vi "1byte.vi"() -> ()   [LabVIEW 2020]
panel:
  out "Actual Bitrate kHz":i32=1000
  out "error out":errorcluster
  in  "SCLK (kHz)":i32=2000 min=0
  out "Cheetah Handle":i32
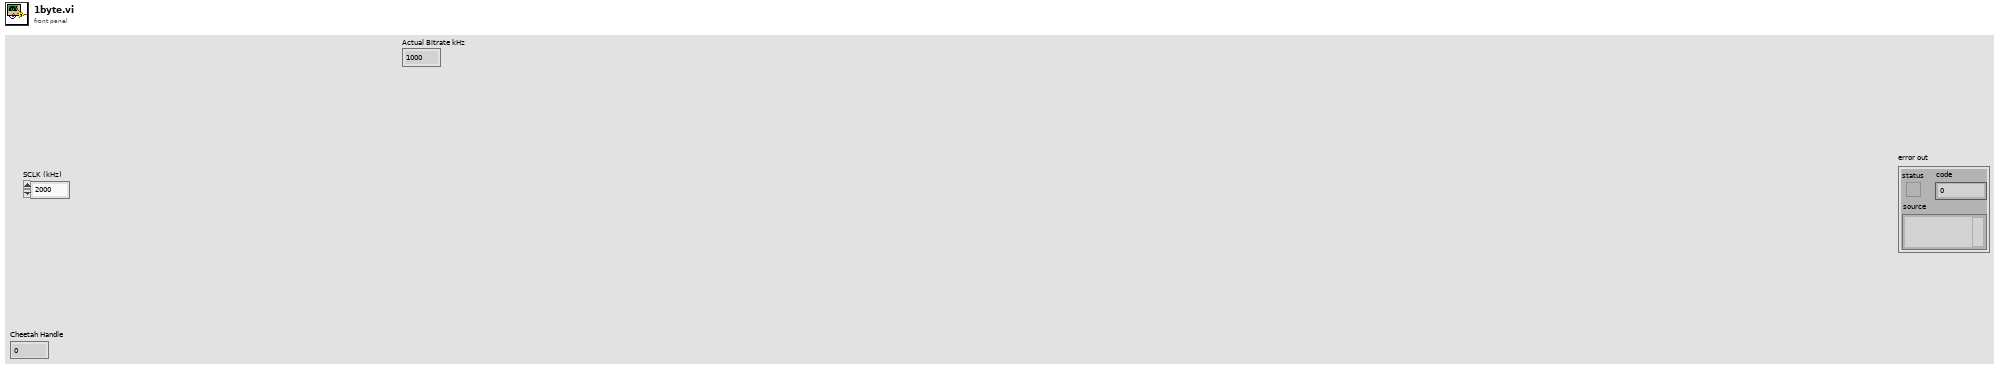
[diagram p1: front panel]
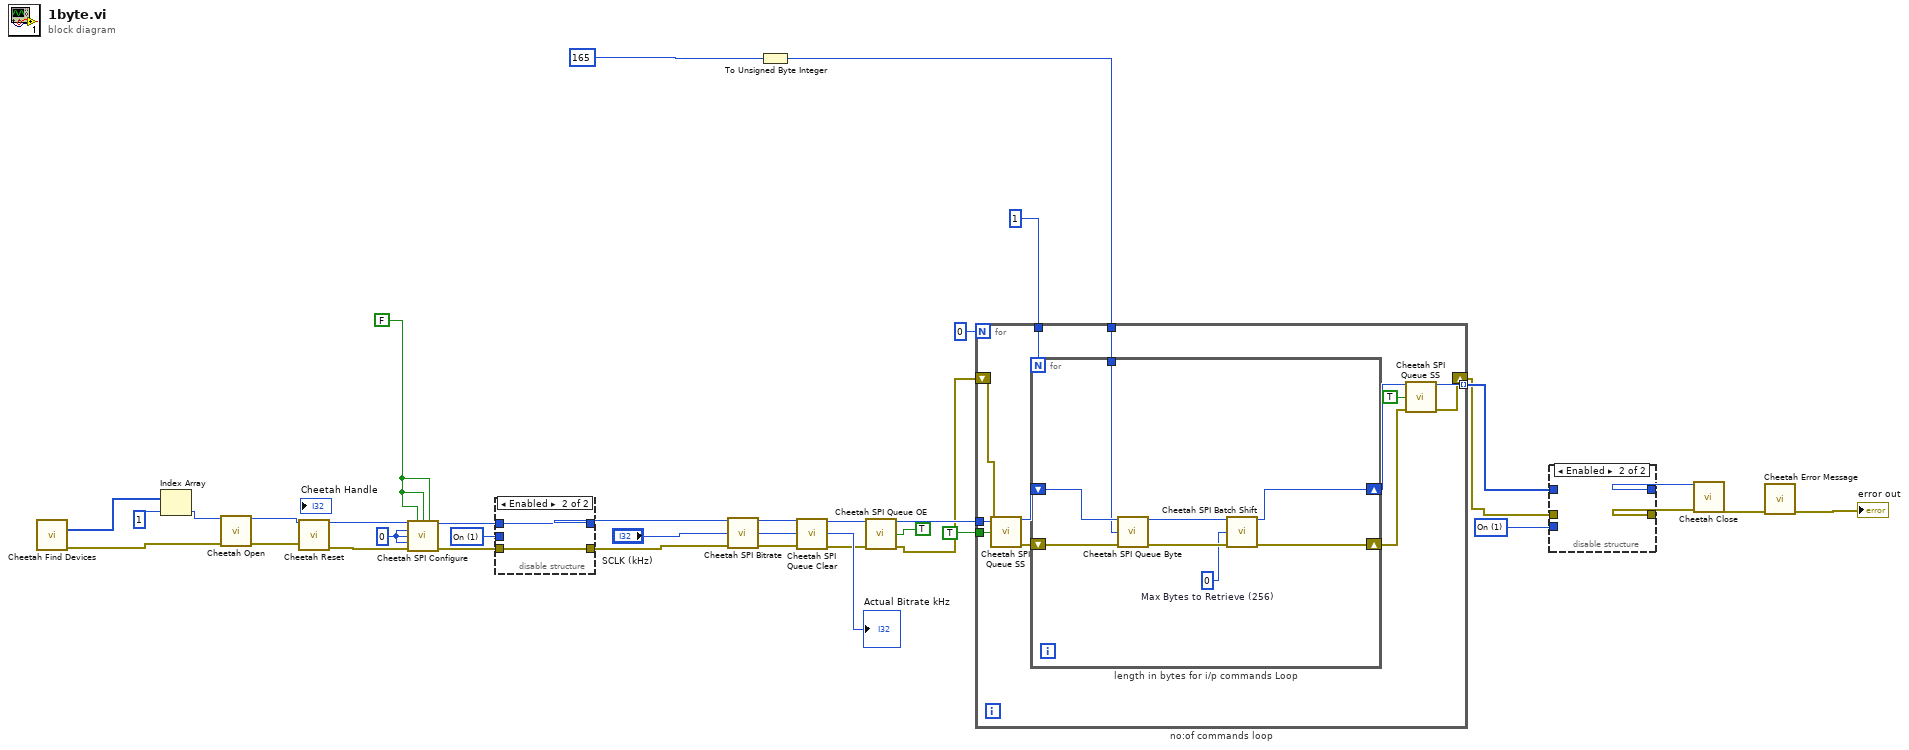
[diagram p0: block diagram]
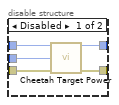
[diagram p2: hidden frame]
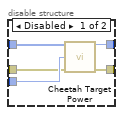
[diagram p3: hidden frame]
diagram:
  w1 = u16 1 items=["Off", "On", "Query"] ("Requested Configuration (2: Query)")
  w22 = u16 1 items=["Off", "On", "Query"] ("Requested Configuration (2: Query)")
  w33 = FALSE
  w34 = 0
  n1 = call <instrlib>:"Cheetah Find Devices.vi"() -> ("Ports"=w35:u16[], "error out"=w10:errorcluster)  [unwired: 13 in, 1 out]
  n2 = Index Array(array=w35, index=1) -> (element=w9:u16)
  n3 = call <instrlib>:"Cheetah Open.vi"("Port Number (0)"=w9, "error in (no error)"=w10) -> ("Cheetah Handle"=w6:i32, "error out"=w7:errorcluster)  [unwired: 12 in]
  n4 = call <instrlib>:"Cheetah Reset.vi"("Cheetah Handle (0)"=w6, "error in (no error)"=w7) -> ("dup Cheetah Handle"=w5:i32, "error out"=w8:errorcluster)  [unwired: 12 in]
  n5 = call <instrlib>:"Cheetah SPI Configure.vi"("Cheetah Handle"=w5, "SS0 Active High? (False)"=w33, "SS1 Active High? (False)"=w33, "SS2 Active High? (False)"=w33, "Polarity (0: Rising/Falling)"=w34, "Phase (0: Sample/Setup)"=w34, "Bitorder (0: MSB)"=w34, "error in (no error)"=w8) -> ("dup Cheetah Handle"=w31:i32, "error out"=w32:errorcluster)  [unwired: 6 in]
  n6 = disable-structure shown="Enabled" {
    disable-tunnel: w32 -> [w41 w42]
    disable-tunnel: w31 -> [w40 w43]
    disable-tunnel: [w39 w42] -> w30
    disable-tunnel: [w38 w43] -> w28
    disable-tunnel: w22 -> [w37 _]
    frame Disabled {
      n7 = call <instrlib>:"Cheetah Target Power.vi"("Cheetah Handle"=w40, "Requested Configuration (2: Query)"=w37, "error in (no error)"=w41) -> ("dup Cheetah Handle"=w38:i32, "error out"=w39:errorcluster)  [unwired: 10 in, 1 out]
    }
    frame Enabled {
    }
  }
  n8 = call <instrlib>:"Cheetah SPI Bitrate.vi"("Cheetah Handle"=w28, "Requested Bitrate kHz (1000)"="SCLK (kHz)", "error in (no error)"=w30) -> ("dup Cheetah Handle"=w27:i32, "Actual Bitrate kHz"=→"Actual Bitrate kHz":i32, "error out"=w26:errorcluster)  [unwired: 10 in]
  n9 = To Unsigned Byte Integer(number=u8 165) -> (unsigned 8bit integer=w13:u8)
  n10 = call <instrlib>:"Cheetah SPI Queue Clear.vi"("Cheetah Handle"=w27, "error in (no error)"=w26) -> ("dup Cheetah Handle"=w21:i32, "error out"=w14:errorcluster)  [unwired: 12 in]
  n11 = call <instrlib>:"Cheetah SPI Queue OE.vi"("Cheetah Handle"=w21, "Output Enable (on)"=TRUE, "error in (no error)"=w14) -> ("dup Cheetah Handle"=w17:i32, "error out"=w15:errorcluster)  [unwired: 11 in]
  n12 = for "no:of commands loop" {
    N: 0 -> [_]
    tunnel: w17 -> [w55]
    tunnel: w13 -> [w51]
    tunnel: 1 -> [w50]
    tunnel: TRUE ("SS1 Assert? (True)") -> [w49]
    shift-right: [w44] -> w3
    shift-left: w15 -> [w54]
    tunnel: [w45] -> w4 mode=indexing
    n13 = call <instrlib>:"Cheetah SPI Queue SS.vi"("Cheetah Handle"=w55, "SS1 Assert? (True)"=w49, "error in (no error)"=w54) -> ("dup Cheetah Handle"=w53:i32, "error out"=w52:errorcluster)  [unwired: 11 in]
    n14 = for "length in bytes for i/p commands Loop" {
      N: w50 -> [_]
      tunnel: w51 -> [w57]
      shift-right: [w59] -> w48
      shift-left: w53 -> [w63]
      shift-right: [w58] -> w46
      shift-left: w52 -> [w62]
      w56 = 0  # Max Bytes to Retrieve (256)
      n15 = call <instrlib>:"Cheetah SPI Queue Byte.vi"("Cheetah Handle"=w63, "Byte Value (0x00)"=w57, "error in (no error)"=w62) -> ("dup Cheetah Handle"=w61:i32, "error out"=w60:errorcluster)  [unwired: 11 in]
      n16 = call <instrlib>:"Cheetah SPI Batch Shift.vi"("Cheetah Handle"=w61, "Max Bytes to Retrieve (256)"=w56, "error in (no error)"=w60) -> ("dup Cheetah Handle"=w59:i32, "error out"=w58:errorcluster)  [unwired: 9 in, 2 out]
    }
    n17 = call <instrlib>:"Cheetah SPI Queue SS.vi"("Cheetah Handle"=w48, "SS1 Assert? (True)"=TRUE, "error in (no error)"=w46) -> ("dup Cheetah Handle"=w45:i32, "error out"=w44:errorcluster)  [unwired: 11 in]
  }
  n18 = disable-structure "Diagram Disable Structure" shown="Enabled" {
    disable-tunnel: [w68 _] -> w25
    disable-tunnel: [w67 _] -> w24
    disable-tunnel: w1 -> [w66 _]
    disable-tunnel: w4 -> [w65 _]
    disable-tunnel: w3 -> [w64 _]
    frame Disabled {
      n19 = call <instrlib>:"Cheetah Target Power.vi"("Cheetah Handle"=w65, "Requested Configuration (2: Query)"=w66, "error in (no error)"=w64) -> ("dup Cheetah Handle"=w68:i32, "error out"=w67:errorcluster)  [unwired: 10 in, 1 out]
    }
    frame Enabled {
    }
  }
  n20 = call <instrlib>:"Cheetah Close.vi"("Cheetah Handle"=w25, "error in (no error)"=w24) -> ("error out"=w23:errorcluster)  [unwired: 12 in, 1 out]
  n21 = call <instrlib>:"Cheetah Error Message.vi"("error in (no error)"=w23) -> ("error out"=→"error out":errorcluster)  [unwired: 10 in, 4 out]
